vi "Show VI FP.vi"(8 "error in (no error)":errorcluster, 11 "Web FP In":refnum<class "Web Front Panel.lvclass">) -> (0 "error out":errorcluster, 3 "Web FP Out":refnum<class "Web Front Panel.lvclass">)   [LabVIEW 2015, in "Front Panel Publisher.lvlib" / "Web Front Panel.lvclass"]
uses:
  Web Front Panel.lvclass
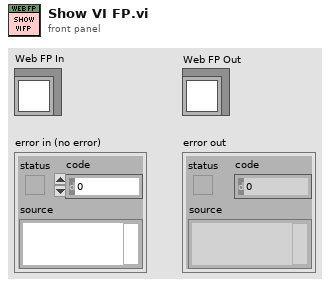
[diagram p1: front panel]
types:
  T1 = enum32{"Invalid", "Standard", "Closed", "Hidden", "Minimized", "Maximized"}
  T2 = typedef "Front Panel Publisher.lvlib/Web Front Panel.lvclass/Object Attributes.ctl" = cluster{"VI Name":string, "VI Reference":refnum<vi>, "Controls":refnum<class "Object.lvclass">[], "Indicators":refnum<class "Object.lvclass">[], "Decorations":refnum<class "Object.lvclass">[], "VR With Previous Get":refnum<data-value>, "VR With Ring Images":refnum<data-value>}
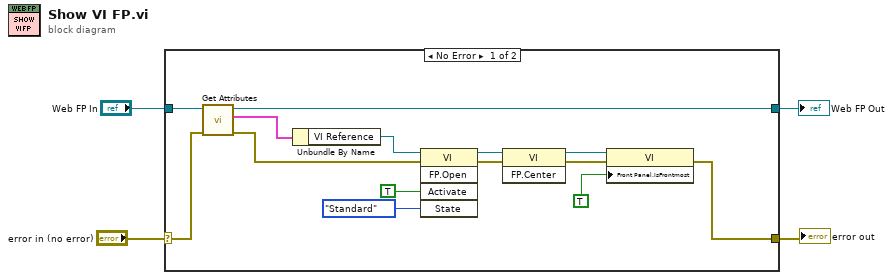
[diagram p0: block diagram]
diagram:
  n1 = case shown="No Error" "error in (no error)" {
    selector: "error in (no error)" -> [w18 w20]
    tunnel: [w5 w20] -> w3
    tunnel: [w15 w19] -> w1
    tunnel: "Web FP In" -> [w16 w19]
    frame No Error {
      n2 = call "Get Attributes.vi"("error in (no error)"=w18, "Web FP In"=w16) -> ("error out"=w6:errorcluster, "Data"=w17:T2, "Web FP Out"=w15:refnum<class "Web Front Panel.lvclass">)  [unwired: 6 in, 1 out]
      n3 = Unbundle By Name(w17) -> ("VI Reference"=w7:refnum<vi>)
      n4 = invoke class="VI" method="FP.Open"(reference=w7, error in=w6, "Activate"=TRUE ("Activate?"), "State"=T1."Standard") -> (reference out=w13:refnum<vi>, error out=w10:errorcluster)  [unwired: 1 in, 3 out]
      n5 = invoke class="VI" method="FP.Center"(reference=w13, error in=w10) -> (reference out=w11:refnum<vi>, error out=w12:errorcluster)  [unwired: 1 in, 1 out]
      n6 = property class="VI"(reference=w11, error in=w12, "Front Panel.IsFrontmost"=TRUE ("Front Panel Window:Is Frontmost")) -> (error out=w5:errorcluster)  [unwired: 1 out]
    }
    frame Error {
    }
  }
  "error out" <- w3
  "Web FP Out" <- w1
